vi "Configure Top and Base Levels.vi"(0 "VISA resource name":refnum<visa-resource-name>, 1 "Base Voltage (5 V)":dbl=5.0, 5 "Channel (15: All Waveforms)":u16(ring)=15 items=["Channel 1"=1, "Channel 2"=2, "Channel 3"=3, "Channel 4"=4, "Function 1"=5, "Function 2"=6, "Function 3"=7, "Function 4"=8, "Memory 1"=9, "Memory 2"=10, "Memory 3"=11, "Memory 4"=12, "All Waveforms"=15], 7 "Deriving Method (0: Absolute)":i32(ring) items=["Absolute", "Histonly", "Minmax", "Standard"], 11 "error in (no error)":errorcluster, 12 "Top Voltage (0 V)":dbl) -> (4 "VISA resource name out":refnum<visa-resource-name>, 15 "error out":errorcluster)   [LabVIEW 2020, in "Agilent 90000 Series.lvlib"]
doc: "Configures the top and base levels."
uses:
  Agilent 90000 Series.lvlib
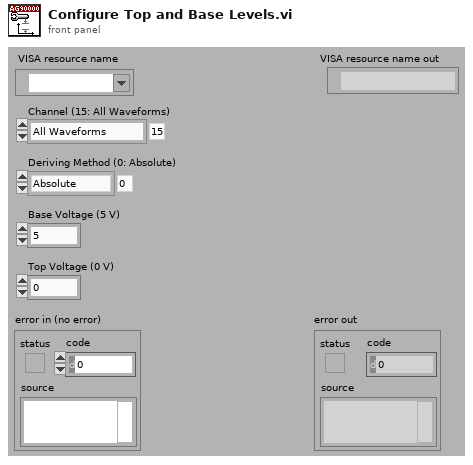
[diagram p1: front panel]
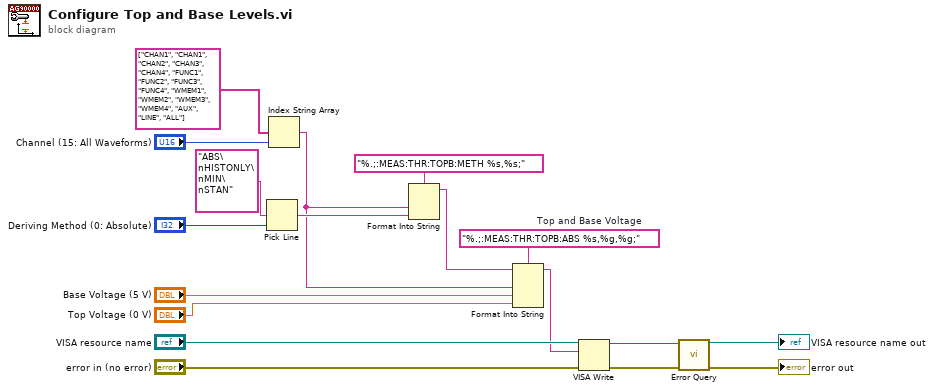
[diagram p0: block diagram]
diagram:
  w18 = "%.;:MEAS:THR:TOPB:ABS %s,%g,%g;"  # Top and Base Voltage
  n1 = Pick Line(multi-line string="ABS\nHISTONLY\nMIN\nSTAN", line index="Deriving Method (0: Absolute)") -> (output string=w7:string)  [unwired: 1 out]
  n2 = Index String Array(1:"Channel (15: All Waveforms)", 2:string[] ["CHAN1", "CHAN1", "CHAN2", "CHAN3", "CHAN4", "FUNC1", "FUNC2", "FUNC3", "FUNC4", "WMEM1", "WMEM2", "WMEM3", "WMEM4", "AUX", "LINE", "ALL"] ("subarray 2")) -> (0:w5:string)  [unwired: 1 out]
  n3 = Format Into String(format string="%.;:MEAS:THR:TOPB:METH %s,%s;", w5, w7) -> (resulting string=w6:string)  [unwired: 2 in, 1 out]
  n4 = Format Into String(format string=w18, initial string=w6, w5, "Base Voltage (5 V)", "Top Voltage (0 V)") -> (resulting string=w2:string)  [unwired: 1 in, 1 out]
  n5 = VISA Write(VISA resource name="VISA resource name", write buffer=w2, error in (no error)="error in (no error)") -> (VISA resource name out=w15:refnum<visa-resource-name>, error out=w14:errorcluster)  [unwired: 1 out]
  n6 = call "Error Query.vi"("error in (no error)"=w14, "VISA resource name"=w15) -> ("error out"=→"error out":errorcluster, "VISA resource name out"=→"VISA resource name out":refnum<visa-resource-name>)  [unwired: 8 out]
